vi "from string.vi"(8 "error in":errorcluster, 9 "data":string, 10 "version":string, 11 "Thermo Channel configuration in":refnum<class "Thermo Channel configuration.lvclass">) -> (0 "error out":errorcluster, 3 "Thermo Channel configuration out":refnum<class "Thermo Channel configuration.lvclass">)   [LabVIEW 2025, in "Thermo.lvlib" / "Thermo Channel configuration.lvclass"]
doc: "Provides an interface for loading a module configuration from a file or other serialized data source. It is recommended that all children of this class store data in two sets--data required for its own initialization, and any data required for parent initialization--and that each implementation uses the <b>Call Parent Method</b> primitive to de-serialize parent information.Copyright 2017 National Instruments Corporation\n\nLicensed under the Apache License, Version 2.0 (the \"License\"); you may not use this file except in compliance with the License. You may obtain a copy of the License at http://www.apache.org/licenses/LICENSE-2.0\nUnless required by applicable law or agreed to in writing, software distributed under the License is distributed on an \"AS IS\" BASIS, WITHOUT WARRANTIES OR CONDITIONS OF ANY KIND, either express or implied. See the License for the specific language governing permissions and limitations under the License."
uses:
  Thermo Channel configuration.lvclass
  Channel Setting.ctl
  Thermo Channel configuration.lvclass/Thermo Channel configuration.ctl
  Users/Public/Documents/Sandia National Labs/TSS Plugin/Abstract Engine.lvlibp/Channel configuration/Channel configuration.lvclass
  Users/Public/Documents/Sandia National Labs/TSS Plugin/CEF.lvlibp/serializable configuration/CEF_serializable configuration.lvclass
  Users/Public/Documents/Sandia National Labs/TSS Plugin/CEF.lvlibp
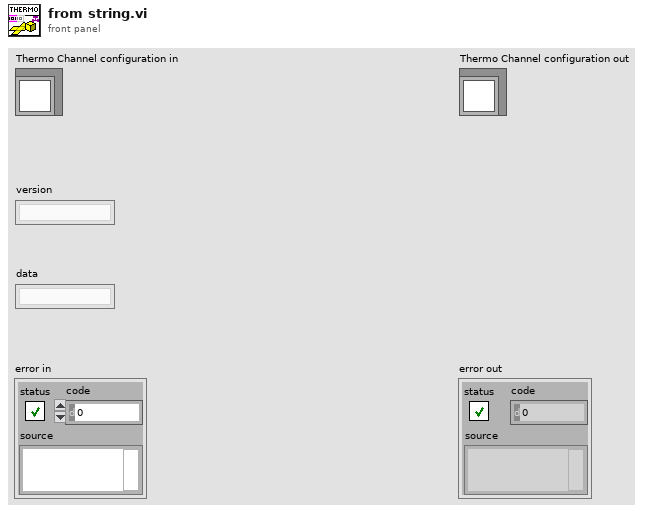
[diagram p1: front panel]
types:
  T1 = typedef "Thermo.lvlib/Thermo Channel configuration.lvclass/Channel Setting.ctl" = cluster{"Numeric":dbl, "Combo":string, "String":string, "Boolean":bool}
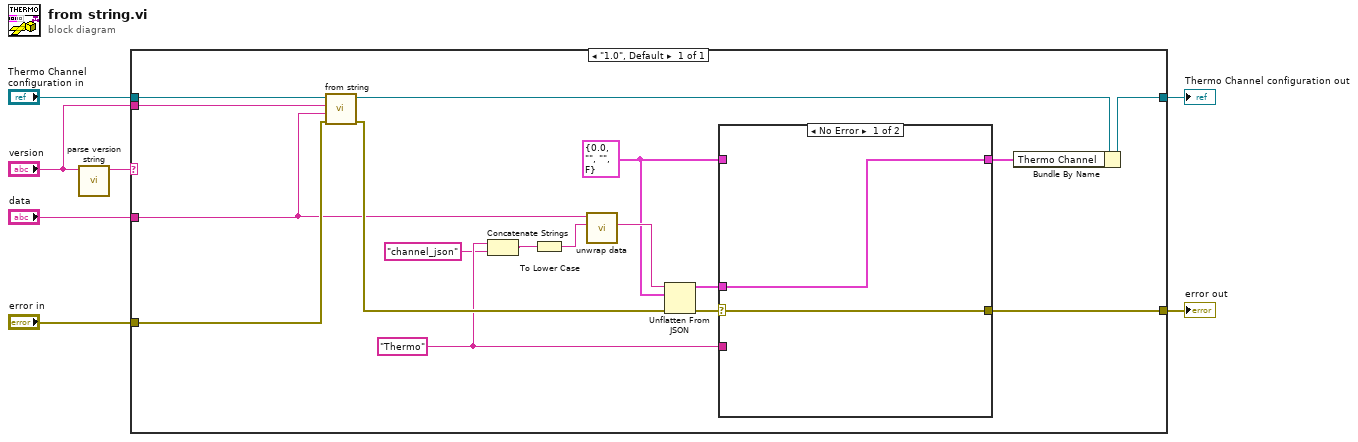
[diagram p0: block diagram]
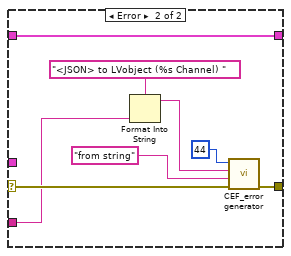
[diagram p2: hidden frame]
diagram:
  n1 = call "parse version string.vi"("full version"="version") -> ("major.minor version"=w3:string)  [unwired: 7 in, 3 out]
  n2 = case shown="\"1.0\", Default" w3 {
    tunnel: "Thermo Channel configuration in" -> [w24]
    tunnel: [w21] -> w6
    tunnel: "data" -> [w16]
    tunnel: "error in" -> [w22]
    tunnel: "version" -> [w20]
    tunnel: [w11] -> w1
    frame "1.0", Default {
      w10 = "Thermo" ("additional identifier")
      w14 = T1 {"Numeric"=0.0, "Combo"="", "String"="", "Boolean"=FALSE} ("Setting")
      n3 = call-parent "from string.vi"("error in"=w22, "data"=w16, "version"=w20, "Channel configuration"=w24) -> ("error out"=w18:errorcluster, "Channel configuration out"=w23:refnum<class "Thermo Channel configuration.lvclass">)  [unwired: 6 in]
      n4 = Concatenate Strings(w10, "channel_json" ("additional identifier")) -> (w8:string)
      n5 = To Lower Case(string=w8) -> (all lower case string=w17:string)
      n6 = call "unwrap data.vi"("identifier"=w17, "data to unwrap"=w16) -> ("unwrapped data"=w15:string)  [unwired: 8 in, 1 out]
      n7 = Unflatten From JSON(JSON string=w15, type and defaults=w14, error in (no error)=w18) -> (value=w12:T1, error out=w13:errorcluster)  [unwired: 4 in]
      n8 = case shown="No Error" w13 {
        selector: w13 -> [w25 w32]
        tunnel: w12 -> [w26 _]
        tunnel: [w26 w31] -> w19
        tunnel: w14 -> [_ w31]
        tunnel: [w25 w30] -> w11
        tunnel: w10 -> [_ w28]
        frame No Error {
        }
        frame Error {
          n9 = Format Into String(format string="<JSON> to LVobject (%s Channel) " ("message"), w28) -> (resulting string=w27:string)  [unwired: 2 in, 1 out]
          n10 = call "CEF_error generator.vi"("error in"=w32, "source"="from string" ("message"), "append error message"=w27, "error code (0)"=44) -> ("error out"=w30:errorcluster)  [unwired: 5 in]
        }
      }
      n11 = Bundle By Name(cluster=w23, "Thermo Channel"=w19) -> (w21:refnum<class "Thermo Channel configuration.lvclass">)
    }
  }
  "error out" <- w1
  "Thermo Channel configuration out" <- w6
